vi "Write dt.vi"(8 "error in (no error)":errorcluster, 10 "dt":dbl, 11 "Data Source in":refnum<class "Data Source.lvclass">) -> (0 "error out":errorcluster, 3 "Data Source out":refnum<class "Data Source.lvclass">)   [LabVIEW 2025]
uses:
  Data Source.lvclass
  C:/Users/natan/Documents/G2CPU-Performance-Demo/Generic Actor/Generic Actor/Generic Actor.lvclass
  C:/Program Files/National Instruments/LabVIEW 2025/vi.lib/MGI/Monitored Actor/Monitored Actor/Monitored Actor/Monitored Actor.lvclass
  C:/Program Files/National Instruments/LabVIEW 2025/vi.lib/ActorFramework/Actor/Actor.lvclass
  C:/Users/natan/Documents/G2CPU-Performance-Demo/Data Source/Data Source/Data Source.lvclass
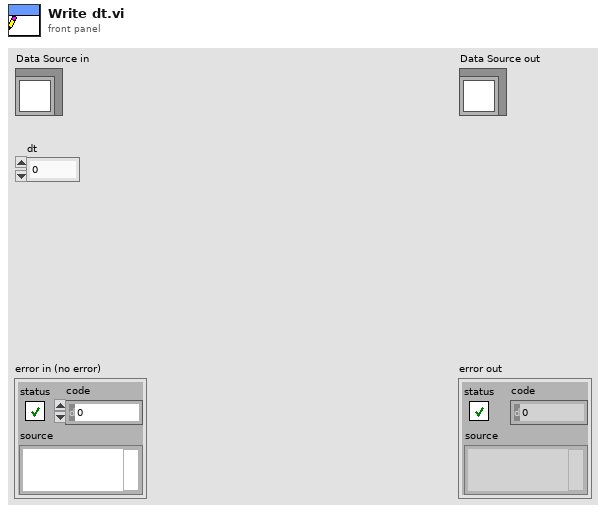
[diagram p1: front panel]
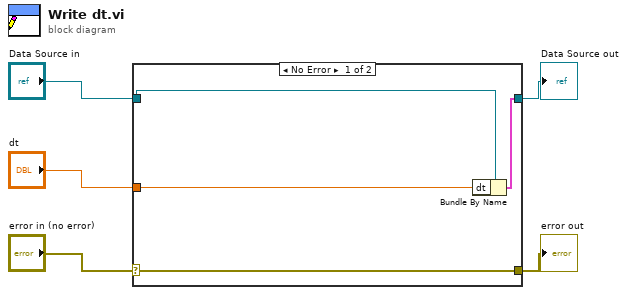
[diagram p0: block diagram]
diagram:
  n1 = case shown="No Error" "error in (no error)" {
    selector: "error in (no error)" -> [w9 w10]
    tunnel: [w9 w10] -> w4
    tunnel: [w7 w11] -> w2
    tunnel: "Data Source in" -> [w8 w11]
    tunnel: "dt" -> [w6 _]
    frame No Error {
      n2 = Bundle By Name(cluster=w8, "dt"=w6) -> (w7:cluster{})
    }
    frame Error {
    }
  }
  "error out" <- w4
  "Data Source out" <- w2
